vi "Test Fail On Specific Error Throwing Expected Error Code.vi"(8 "error in (no error)":errorcluster, 11 "Test Case In":refnum<class "Advanced Asseritions Test.lvclass">) -> (0 "error out":errorcluster, 3 "Test Case Out":refnum<class "Advanced Asseritions Test.lvclass">)   [LabVIEW 2020, in "Advanced Asseritions Test.lvclass"]
uses:
  Advanced Asseritions Test.lvclass
  Advanced Asseritions Test.lvclass/Advanced Asseritions Test.ctl
  e8c5eeff-a694-4c0d-b261-74e2e6f5327d.vi
  source/LUnit Test Case.lvclass
  source/Core/Result/Status.ctl
  source/Core/Result/Result.lvlib
  Test Doubles/Test Case Test Double/Test Case Test Double.lvclass
  Test Doubles/Test Case Test Double/Methods.ctl
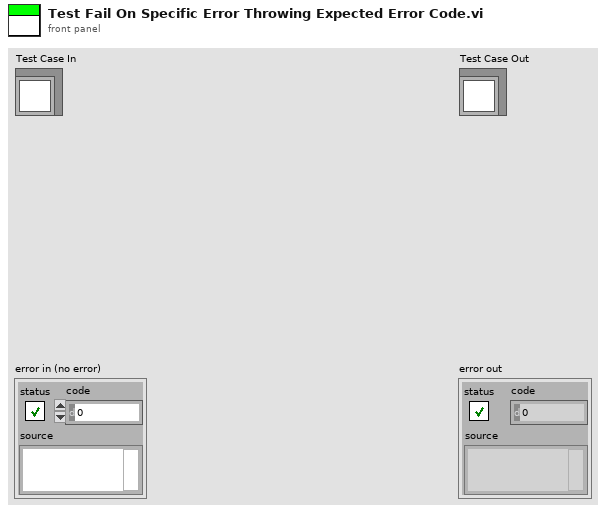
[diagram p1: front panel]
types:
  T1 = typedef "Test Case Test Double.lvclass/Methods.ctl" = enum16{"Test Failing Test.vi", "Test Passing Test.vi", "Test Error Test.vi", "Test Skip Test.vi", "Test Passing Pass If Test.vi", "Test Failing Pass If Test.vi", "Test Failing Fail If Test.vi", "Test Passing Fail If Test.vi", "Test Passing Pass If Error Test.vi", "Test Failing Pass If Error Test.vi", "Test Passing Fail If Error Test.vi", "Test Failing Fail If Error Test.vi", "Test Passing Pass If Equal Test.vi", "Test Failing Pass If Equal Test.vi", "Test Failing Fail If Equal Test.vi", "Test Passing Fail If Equal Test.vi", "Freezing Test.vi", "Test Pass on Expected Error Code.vi", "Test Error on Unexpected Error Code.vi", "Test Fail on Expected Error Code.vi", "Test Error when Fail on Unexpected Error Code.vi", "Test Pass on Expected Element in Array.vi", "Test Fail on Expected Element Not in Array.vi", "Test Pass on Expected Element in Set.vi", "Test Fail on Expected Element Not in Set.vi", "Test Pass on Expected Element in Map.vi", "Test Fail on Expected Element Not in Map.vi", "Test Fail on Unexpected Element in Array.vi", "Test Pass on Unexpected Element Not in Array.vi", "Test Fail if Unexpected Element in Set.vi", "Test Pass if Unexpected Element Not in Set.vi", "Test Fail if Unexpected Element in Map.vi", "Test Pass if Unexpected Element Not in Map.vi", "Test Pass on Expected Element in Array of Clusters.vi", "Test Pass on Expected Element Not in Array of Clusters.vi", "Test Matching String Test.vi", "Test Not Matching String Test.vi", "Verify Passing.vi", "Without Prefix.vi", "Private VI.vi"}
  T2 = typedef "Result.lvlib/Status.ctl" = enum16{"", "Passed", "Failed", "Error", "Skipped", "Setup Error", "Broken", "Teardown Error"}
  T3 = typedef "Result.lvlib/Result.ctl" = cluster{"Name":string, "Description":string, "Status":T2, "Result Type":T4, "Execution Time":dbl, "Data":cluster{"Expected":variant, "Actual":variant, "Delta":variant}}
  T4 = typedef "Result.lvlib/Type.ctl" = enum16{"Test Case", "Test Suite", "Test Run", "Pass", "Fail", "Skip", "Pass if", "Fail if", "Pass if Error", "Fail if Error", "Pass if Equal", "Fail if Equal"}
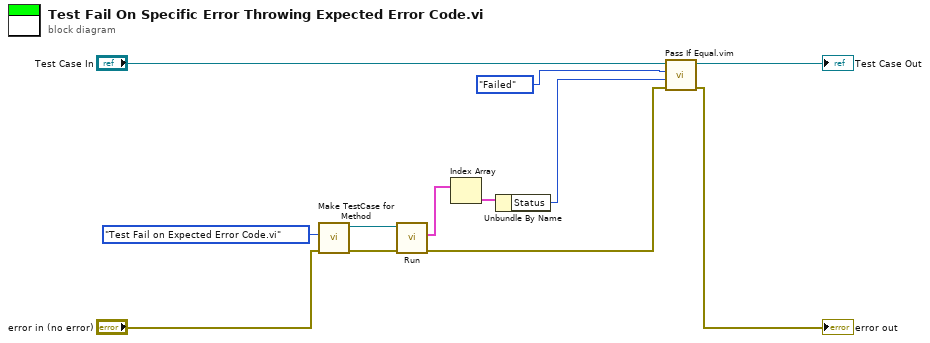
[diagram p0: block diagram]
diagram:
  n1 = call "Make TestCase for Method.vi"("error in (no error)"="error in (no error)", "Test Method"=Methods."Test Fail on Expected Error Code.vi") -> ("error out"=w8:errorcluster, "LUnit Test Case V2 out"=w9:refnum<class "LUnit Test Case.lvclass">)  [unwired: 8 in]
  n2 = call-dynamic "Run.vi"("error in (no error)"=w8, "LUnit Test Case In"=w9) -> ("error out"=w6:errorcluster, "Results"=w5:T3[])  [unwired: 6 in, 2 out]
  n3 = Index Array(array=w5) -> (element=w4:T3)  [unwired: 1 in]
  n4 = Unbundle By Name(w4) -> ("Status"=w3:T2)
  n5 = call "Pass If Equal.vim"("error in (no error)"=w6, "Actual"=w3, "Expected"=Status."Failed" ("Status"), "LUnit Test Case In"="Test Case In") -> ("error out"=→"error out":errorcluster, "LUnit Test Case Out"=→"Test Case Out":refnum<class "Advanced Asseritions Test.lvclass">)  [unwired: 6 in]
